vi "ArrayOfDropletDBs-GFV.vi"(8 "error in (no error)":errorcluster, 9 "DB Name":string, 10 "?":T1=enum."AddDropletDB", 11 "Data in":variant) -> (0 "error out":errorcluster, 3 "Data out":variant)   [LabVIEW 2013]
doc: "Use this template to build a VI to use as a subVI."
uses:
  ArrayofDropletsDBEnum.ctl
  DropletDB.ctl
  TypeDef/MultipleFileData.ctl
  TypeDef/DropletDBListBox.ctl
  ArrayOfDropletDB.ctl
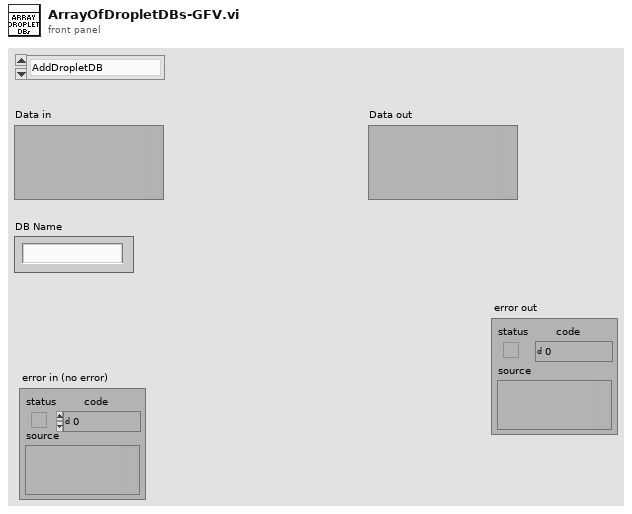
[diagram p1: front panel]
types:
  T1 = typedef "ArrayofDropletsDBEnum.ctl" = enum16{"AnalyzeDropletDBs", "PrepareDBforSave", "GetDBtoListBox", "UpdateDBtoListBox", "AddDBtoListBox", "AddDropletDB", "InitArrayOfDropletDB"}
  T2 = typedef "DropletDBListBox.ctl" = cluster{"DB Name":string, "Include DB":bool}[]
  T3 = typedef "MultipleFileData.ctl" = cluster{"FreezeTemperature":dbl, "FreezeFileInformation":string, "Diameter (microns)":dbl}[]
  T4 = typedef "ArrayOfDropletDB.ctl" = cluster{"DropletArray":cluster{"ImageFreezeIndex":i32, "DropIndex":i32, "Position":cluster{"x":sgl, "y":sgl}, "Bounding Box":cluster{"x":sgl, "y":sgl}[], "Score":sgl, "GreyLevelInBoundingBox":dbl[], "GLDifference":dbl[], "Baseline level":dbl, "Peak":cluster{"Value":dbl, "Index":u32}, "Peak Onset":cluster{"Value":dbl, "Index":u32}, "FreezeFileName":string, "FreezeAbsTime":timestamp, "FreezeTemperature":dbl, "ImageIndexArray":u32[], "Freeze Point Found":bool, "Baseline std":dbl, "FreezedImageArray":cluster{"Image":u8[][]}[], "Include Droplet":bool, "Remark":string, "Freeze Rel Time":u32[], "Diameter (microns)":dbl}[]}[]
  T5 = typedef "DropletDB.ctl" = cluster{"ImageFreezeIndex":i32, "DropIndex":i32, "Position":cluster{"x":sgl, "y":sgl}, "Bounding Box":cluster{"x":sgl, "y":sgl}[], "Score":sgl, "GreyLevelInBoundingBox":dbl[], "GLDifference":dbl[], "Baseline level":dbl, "Peak":cluster{"Value":dbl, "Index":u32}, "Peak Onset":cluster{"Value":dbl, "Index":u32}, "FreezeFileName":string, "FreezeAbsTime":timestamp, "FreezeTemperature":dbl, "ImageIndexArray":u32[], "Freeze Point Found":bool, "Baseline std":dbl, "FreezedImageArray":cluster{"Image":u8[][]}[], "Include Droplet":bool, "Remark":string, "Freeze Rel Time":u32[], "Diameter (microns)":dbl}[]
  T6 = cluster{"Min Diameter (microns)":dbl, "Max Diameter (microns)":dbl}
  T7 = cluster{"FreezeTemperature":dbl, "FreezeFileInformation":string, "Diameter (microns)":dbl}
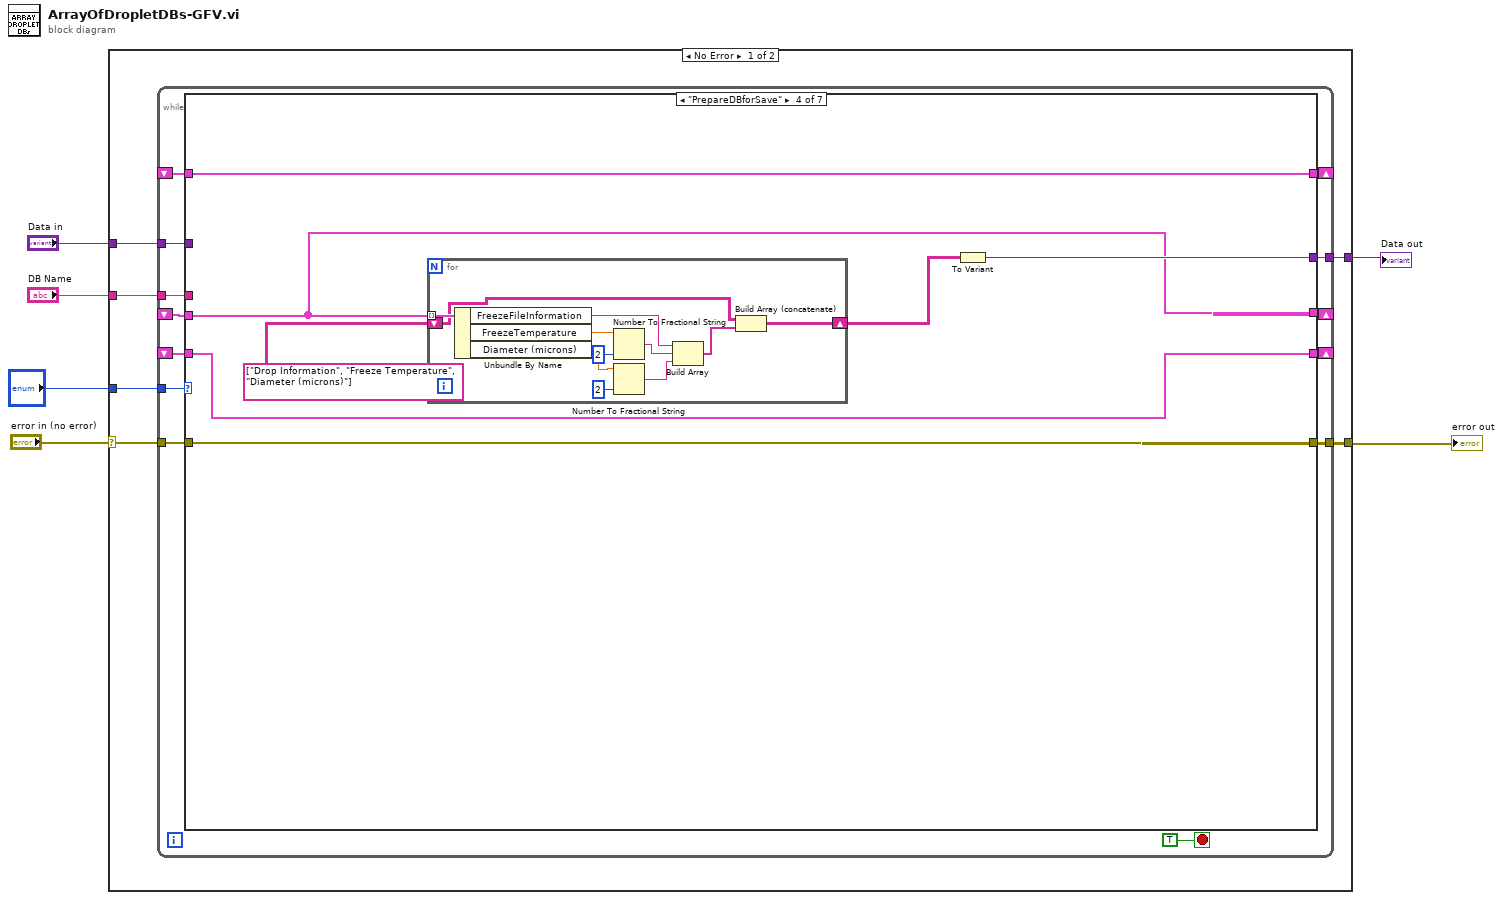
[diagram p0: block diagram]
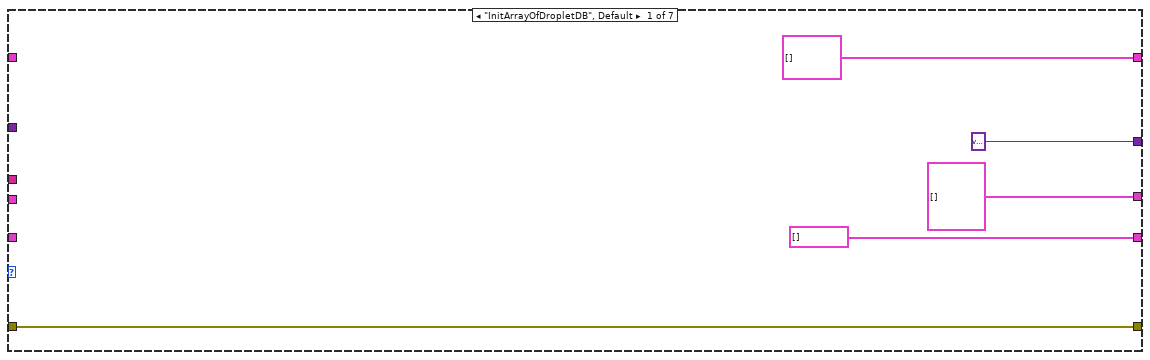
[diagram p2: hidden frame]
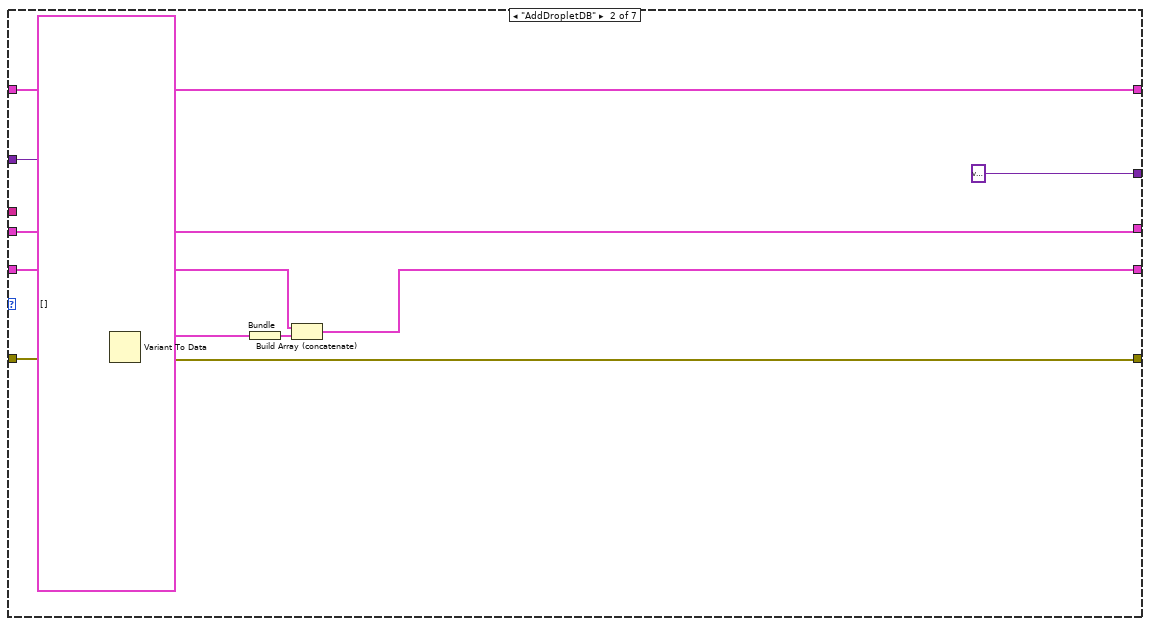
[diagram p3: hidden frame]
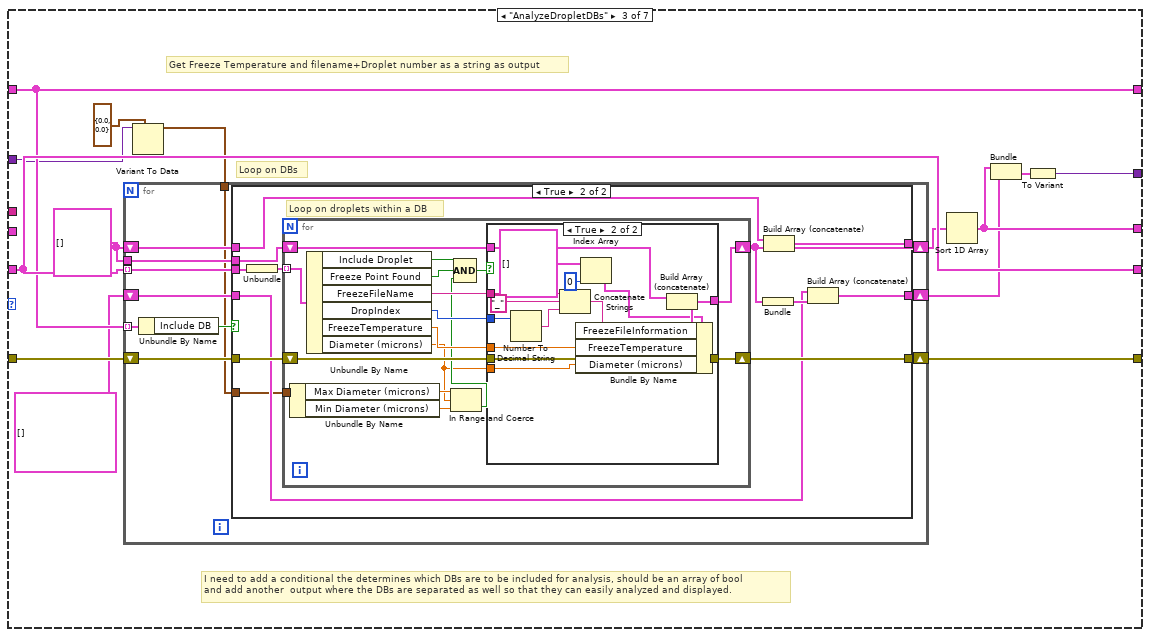
[diagram p4: hidden frame]
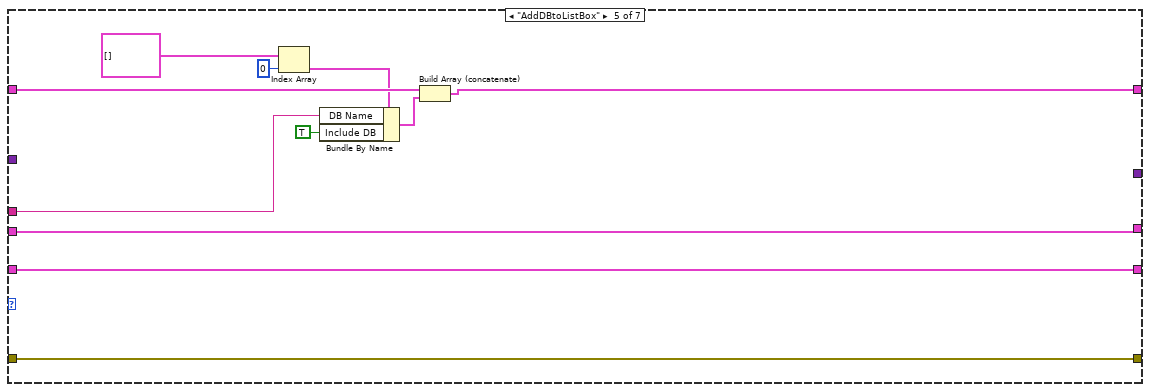
[diagram p7: hidden frame]
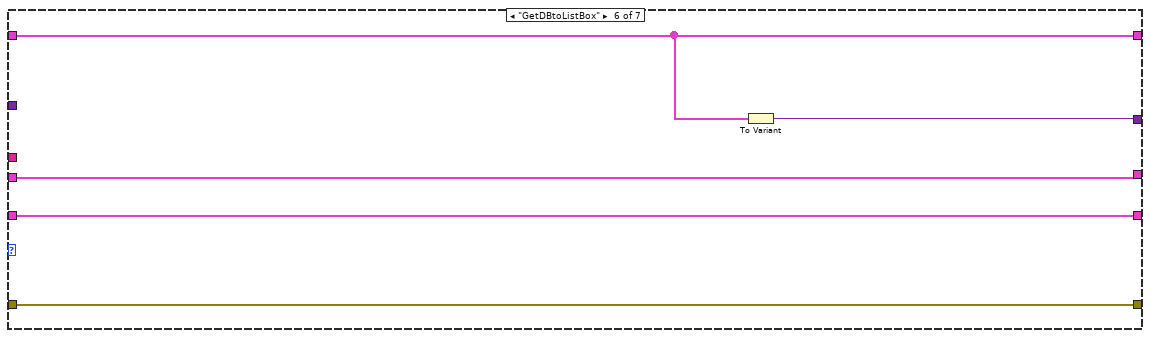
[diagram p8: hidden frame]
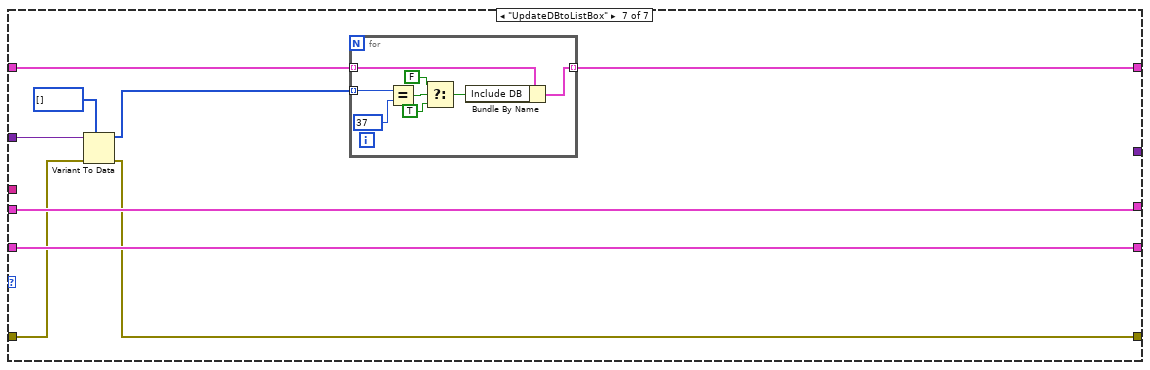
[diagram p9: hidden frame]
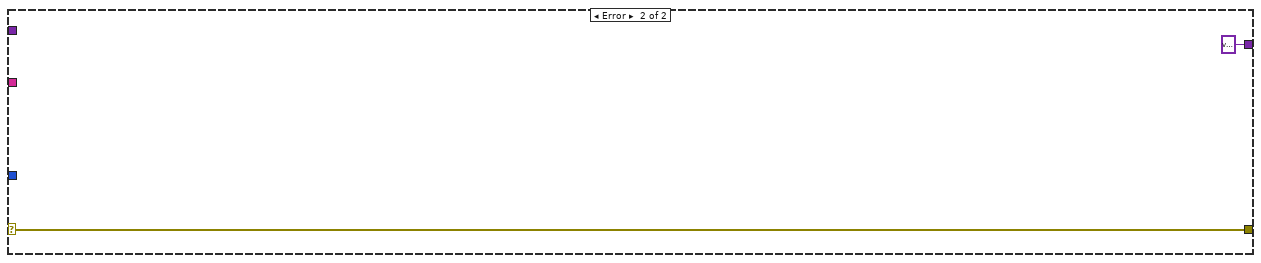
[diagram p10: hidden frame]
diagram:
  n1 = case shown="No Error" "error in (no error)" {
    selector: "error in (no error)" -> [w10 w166]
    tunnel: [w11 w166] -> w5
    tunnel: "?" -> [w12 _]
    tunnel: "Data in" -> [w9 _]
    tunnel: [w8 variant ("Variant")] -> w2
    tunnel: "DB Name" -> [w7 _]
    frame No Error {
      n2 = while {
        tunnel: w12 -> [w24]
        shift-right: [w23] -> _
        shift-left: _ -> [w19]
        tunnel: [w22] -> w11
        tunnel: w10 -> [w21]
        tunnel: w9 -> [w20]
        tunnel: [w18] -> w8
        shift-right: [w17] -> _
        shift-left: _ -> [w16]
        tunnel: w7 -> [w15]
        shift-right: [w14] -> _
        shift-left: _ -> [w13]
        stop <- TRUE stop-if-true
        n3 = case shown="\"PrepareDBforSave\"" w24 {
          tunnel: [T4 [] ("Array of Droplets DB") w36 w53 w116 w140 w147 w156] -> w23
          tunnel: [w29 w34 w54 w117 w141 w145 w148] -> w22
          tunnel: w21 -> [w29 w35 w55 w117 w141 w145 w153]
          tunnel: w20 -> [_ w41 w43 _ _ _ w154]
          tunnel: w19 -> [_ w37 w53 w116 w140 w147 w156]
          tunnel: [variant ("Variant") variant ("Variant") w52 w119 _ w143 _] -> w18
          tunnel: [T3 [] w32 w47 w115 w142 w146 w155] -> w17
          tunnel: w16 -> [_ w32 _ w115 w142 w146 w155]
          tunnel: w15 -> [_ _ _ _ w137 _ _]
          tunnel: [T2 [] ("DropletDBListBoxCtl") w31 w50 w114 w138 w144 w150] -> w14
          tunnel: w13 -> [_ w31 w50 w114 w139 w144 w151]
          frame "InitArrayOfDropletDB", Default {
          }
          frame "AddDropletDB" {
            n4 = Variant To Data(error in=w35, type=T5 [] ("DropletArray"), Variant=w41) -> (data=w39:T5, error out=w34:errorcluster)
            n5 = Bundle("DropletArray"=w39) -> (w38:cluster{"DropletArray":T5})  [unwired: 1 in]
            n6 = Build Array (concatenate)(w37, w38) -> (w36:cluster{"DropletArray":T5}[])
          }
          frame "AnalyzeDropletDBs" {
            w49 = T3 []
            # "I need to add a conditional the determines which DBs are to be included for analysis, should be an array of bool\nand add another  output where the DBs are separated as well so that they can easily analyzed and displayed."
            # "Get Freeze Temperature and filename+Droplet number as a string as output"
            # "Loop on DBs"
            n7 = Variant To Data(type=T6 {"Min Diameter (microns)"=0.0, "Max Diameter (microns)"=0.0} ("output cluster"), Variant=w43) -> (data=w42:T6)  [unwired: 1 in, 1 out]
            n8 = for {
              tunnel: w53 -> [w64] mode=indexing
              shift-right: [w65] -> w54
              shift-left: w55 -> [w66]
              shift-right: [w63] -> w51
              shift-left: w49 -> [w62]
              tunnel: w49 -> [w61]
              tunnel: w50 -> [w60] mode=indexing
              shift-right: [w58] -> w46
              shift-left: cluster{T3}[] [] -> [w57]
              tunnel: w42 -> [w56]
              n9 = Unbundle By Name(w60) -> ("Include DB"=w59:bool)
              n10 = case shown="True" w59 {
                tunnel: w66 -> [w69 w81]
                tunnel: [w69 w80] -> w65
                tunnel: w64 -> [_ w79]
                tunnel: [w68 w77] -> w63
                tunnel: w62 -> [w68 w76]
                tunnel: w61 -> [_ w75]
                tunnel: [w67 w72] -> w58
                tunnel: w57 -> [w67 w71]
                tunnel: w56 -> [_ w70]
                frame False {
                }
                frame True {
                  # "Loop on droplets within a DB"
                  n11 = Unbundle(w79) -> ("DropletArray"=w78:T5)
                  n12 = for {
                    shift-right: [w91] -> w80
                    shift-left: w81 -> [w90]
                    tunnel: w78 -> [w97] mode=indexing
                    shift-right: [w93] -> w74
                    shift-left: w75 -> [w92]
                    tunnel: w70 -> [w89]
                    n13 = Unbundle By Name(w89) -> ("Max Diameter (microns)"=w88:dbl, "Min Diameter (microns)"=w87:dbl)
                    n14 = Unbundle By Name(w97) -> ("Include Droplet"=w85:bool, "Freeze Point Found"=w84:bool, "FreezeFileName"=w96:string, "DropIndex"=w95:i32, "FreezeTemperature"=w94:dbl, "Diameter (microns)"=w82:dbl)
                    n15 = In Range and Coerce(upper limit=w88, x=w82, lower limit=w87) -> (In Range?=w86:bool)  [unwired: 1 out]
                    n16 = Compound Arithmetic op=AND(w85, w84, w86) -> (w83:bool)
                    n17 = case shown="True" w83 {
                      tunnel: w96 -> [_ w113]
                      tunnel: w95 -> [_ w111]
                      tunnel: w94 -> [_ w108]
                      tunnel: [w99 w106] -> w93
                      tunnel: w92 -> [w99 w105]
                      tunnel: [w98 w104] -> w91
                      tunnel: w90 -> [w98 w104]
                      tunnel: w82 -> [_ w100]
                      frame False {
                      }
                      frame True {
                        n18 = Number To Decimal String(number=w111) -> (decimal integer string=w110:string)  [unwired: 1 in]
                        n19 = Concatenate Strings(w113, "_" ("string"), w110) -> (w109:string)
                        n20 = Index Array(array=T3 [] ("Array"), index=0) -> (element=w101:T7)
                        n21 = Bundle By Name(cluster=w101, "FreezeFileInformation"=w109, "FreezeTemperature"=w108, "Diameter (microns)"=w100) -> (w107:T7)
                        n22 = Build Array (concatenate)(w105, w107) -> (w106:T3)
                      }
                    }
                  }
                  n23 = Bundle(w74) -> (w73:cluster{T3})  [unwired: 1 in]
                  n24 = Build Array (concatenate)(w76, w74) -> (w77:T3)
                  n25 = Build Array (concatenate)(w71, w73) -> (w72:cluster{T3}[])
                }
              }
            }
            n26 = Sort 1D Array(array=w51) -> (sorted array=w47:T3)
            n27 = Bundle(w47, w46) -> (w45:cluster{T3, cluster{T3}[]})  [unwired: 1 in]
            n28 = To Variant(anything=w45) -> (Variant=w52:variant)
          }
          frame "PrepareDBforSave" {
            n29 = for {
              tunnel: w115 -> [w131] mode=indexing
              shift-right: [w128] -> w118
              shift-left: string[][] [["Drop Information", "Freeze Temperature", "Diameter (microns)"]] -> [w127]
              n30 = Unbundle By Name(w131) -> ("FreezeFileInformation"=w126:string, "FreezeTemperature"=w130:dbl, "Diameter (microns)"=w122:dbl)
              n31 = Number To Fractional String(number=w130, precision (6)=i16 2) -> (F-format string=w125:string)  [unwired: 2 in]
              n32 = Number To Fractional String(number=w122, precision (6)=i16 2) -> (F-format string=w121:string)  [unwired: 2 in]
              n33 = Build Array(w126, w125, w121) -> (w124:string[])
              n34 = Build Array (concatenate)(w127, w124) -> (w128:string[][])
            }
            n35 = To Variant(anything=w118) -> (Variant=w119:variant)
          }
          frame "AddDBtoListBox" {
            n36 = Index Array(array=T2 [] ("DropletDBListBoxCtl"), index=0) -> (element=w134:cluster{"DB Name":string, "Include DB":bool})
            n37 = Bundle By Name(cluster=w134, "DB Name"=w137, "Include DB"=TRUE) -> (w132:cluster{"DB Name":string, "Include DB":bool})
            n38 = Build Array (concatenate)(w139, w132) -> (w138:T2)
          }
          frame "GetDBtoListBox" {
            n39 = To Variant(anything=w144) -> (Variant=w143:variant)
          }
          frame "UpdateDBtoListBox" {
            n40 = Variant To Data(error in=w153, type=i32[] [] ("output array"), Variant=w154) -> (data=w149:i32[], error out=w148:errorcluster)
            n41 = for {
              tunnel: w151 -> [w164] mode=indexing
              tunnel: [w163] -> w150 mode=indexing
              tunnel: w149 -> [w158] mode=indexing
              n42 = Equal?(x=w158, y=37 ("Item Symbols")) -> (x = y?=w162:bool)
              n43 = Select(t=FALSE, s=w162, f=TRUE) -> (s? t:f=w161:bool)
              n44 = Bundle By Name(cluster=w164, "Include DB"=w161) -> (w163:cluster{"DB Name":string, "Include DB":bool})
            }
          }
        }
      }
    }
    frame Error {
    }
  }
  "error out" <- w5
  "Data out" <- w2
